vi "Write Channel suffix.vi"(8 "error in (no error)":errorcluster, 10 "Channel suffix":string, 11 "Tag Channel Column in":refnum<class "Tag Channel Column.lvclass">) -> (0 "error out":errorcluster, 3 "Tag Channel Column out":refnum<class "Tag Channel Column.lvclass">)   [LabVIEW 2013, in "Table Manager.lvlib" / "Tag Channel Column.lvclass"]
uses:
  Tag Channel Column.lvclass
  Tag Channel Column.lvclass/Tag Channel Column.ctl
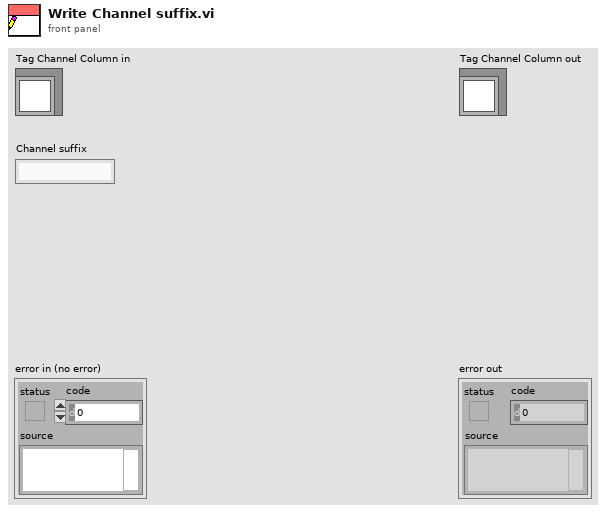
[diagram p1: front panel]
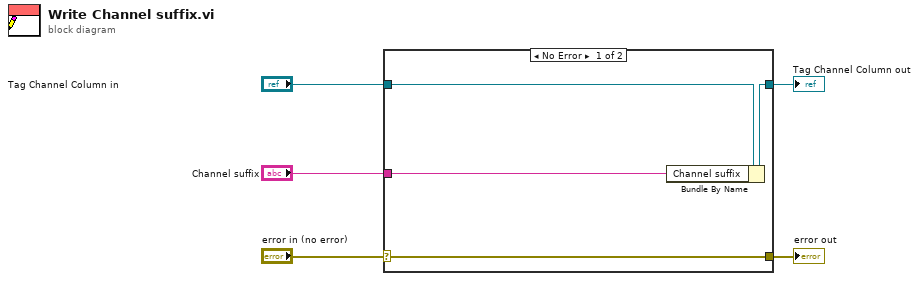
[diagram p0: block diagram]
diagram:
  n1 = case shown="No Error" "error in (no error)" {
    selector: "error in (no error)" -> [w9 w10]
    tunnel: [w9 w10] -> w4
    tunnel: [w7 w11] -> w2
    tunnel: "Tag Channel Column in" -> [w8 w11]
    tunnel: "Channel suffix" -> [w6 _]
    frame No Error {
      n2 = Bundle By Name(cluster=w8, "Channel suffix"=w6) -> (w7:refnum<class "Tag Channel Column.lvclass">)
    }
    frame Error {
    }
  }
  "error out" <- w4
  "Tag Channel Column out" <- w2
